vi "120_cm_Scoring.vi"() -> (0 "String":string, 3 "Cluster":cluster{"State":T1, "Drive Control":T2} {"Drive Control"."Power (100)" min=-100 max=100})   [LabVIEW 2012, in "Serenity_mk2.lvrbt"]
uses:
  Serenity_mk2.lvrbt
  State_Typ.ctl
  auto_drive_TYP.ctl
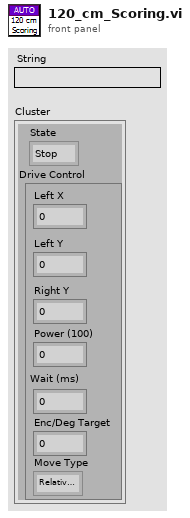
[diagram p1: front panel]
types:
  T1 = typedef "State_Typ.ctl" = enum16{"Stop", "Check for Position 3", "Check for Position 2", "Move", "Reset Enc", "Read Enc", "Lift", "Dump Close"}
  T2 = typedef "auto_drive_TYP.ctl" = cluster{"Left X":i8, "Left Y":i8, "Right Y":i8, "Power (100)":i8, "Wait (ms)":u32, "Enc/Deg Target":i32, "Move Type":enum16{"Relative Degrees", "Wait", "Encoder"}}
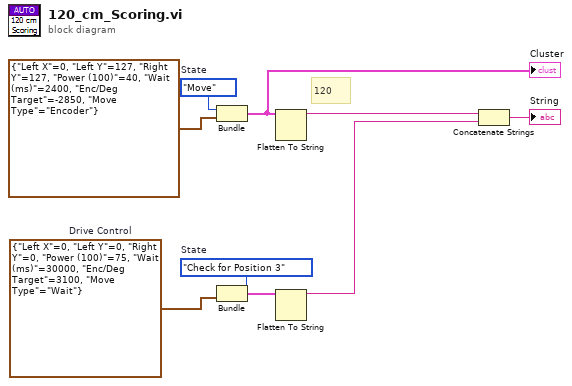
[diagram p0: block diagram]
diagram:
  w6 = T2 {"Left X"=0, "Left Y"=0, "Right Y"=0, "Power (100)"=75, "Wait (ms)"=30000, "Enc/Deg Target"=3100, "Move Type"=enum."Wait"}  # Drive Control
  w5 = State_Typ."Check for Position 3"  # State
  w2 = State_Typ."Move"  # State
  # "120"
  n1 = Bundle("State"=w2, "Drive Control"=T2 {"Left X"=0, "Left Y"=127, "Right Y"=127, "Power (100)"=40, "Wait (ms)"=2400, "Enc/Deg Target"=-2850, "Move Type"=enum."Encoder"}) -> (w8:cluster{"State":T1, "Drive Control":T2})  [unwired: 1 in]
  "Cluster" <- w8
  n2 = Bundle("State"=w5, "Drive Control"=w6) -> (w4:cluster{"State":T1, "Drive Control":T2})  [unwired: 1 in]
  n3 = Flatten To String(anything=w8) -> (data string=w3:string)  [unwired: 3 in, 2 out]
  n4 = Flatten To String(anything=w4) -> (data string=w7:string)  [unwired: 3 in, 2 out]
  n5 = Concatenate Strings(w3, w7) -> (→"String":string)
